vi "upload dir.vi"() -> ()   [LabVIEW 2010]
uses:
  <vilib>/addons/database/Connection.llb/DB Tools Open Connec (Path).vi
  <vilib>/addons/database/NI_Database_API.lvlib
panel:
  out "Slide":dbl(slide) scale=0.0..1.0
  in  "UDL":path=path "D:/Ab-initio/VASP Calcs/VASP DB.udl"
  in  "Primary Path":path
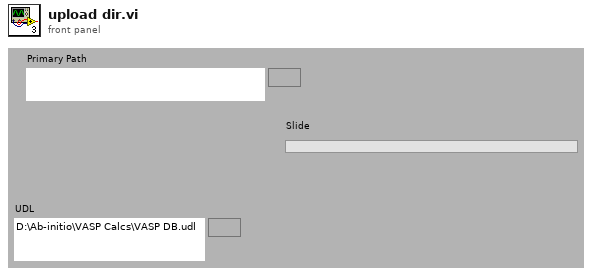
[diagram p1: front panel]
types:
  T1 = typedef "NI_Database_API.lvlib/Conn ObjectReference.ctl" = refnum<k1>
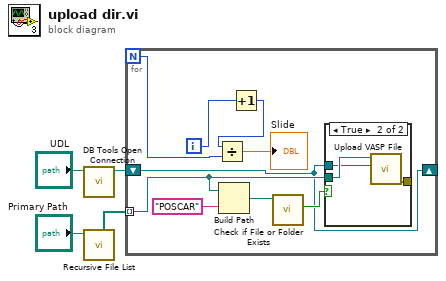
[diagram p0: block diagram]
diagram:
  n1 = call-poly <vilib>:"DB Tools Open Connection.vi"("connection information"="UDL") -> ("connection reference"=w1:T1)  [unwired: 7 in, 1 out]
  n2 = call <vilib>:"Recursive File List.vi"("Folder Path"="Primary Path") -> ("All Folders"=w3:path[])  [unwired: 6 in, 4 out]
  n3 = for {
    N -> [w8]
    tunnel: w3 -> [w10] mode=indexing
    shift-right: [w9] -> _
    shift-left: w1 -> [w9]
    i -> [w6]
    n4 = Build Path(base path=w10, name or relative path="POSCAR") -> (appended path=w12:path)
    n5 = Increment(x=w6) -> (x+1=w5:i32)
    n6 = Divide(x=w5, y=w8) -> (x/y=→"Slide":dbl)
    n7 = call <vilib>:"Check if File or Folder Exists.vi"("path"=w12) -> ("file or folder exists?"=w11:bool)  [unwired: 8 in, 2 out]
    n8 = case shown="True" w11 {
      tunnel: w10 -> [_ w16]
      tunnel: w9 -> [_ w15]
      tunnel: [_ w14] -> _
      frame False {
      }
      frame True {
        n9 = call "Upload VASP File.vi"("connection reference"=w15, "Directory to upload"=w16) -> ("error out"=w14:errorcluster)  [unwired: 8 in, 1 out]
      }
    }
  }
